vi "init queues.vi"(8 "error in (no error)":errorcluster) -> (0 "error out":errorcluster, 3 "output device queues":T1)   [LabVIEW 2016]
uses:
  data.ctl
  device/device.ctl
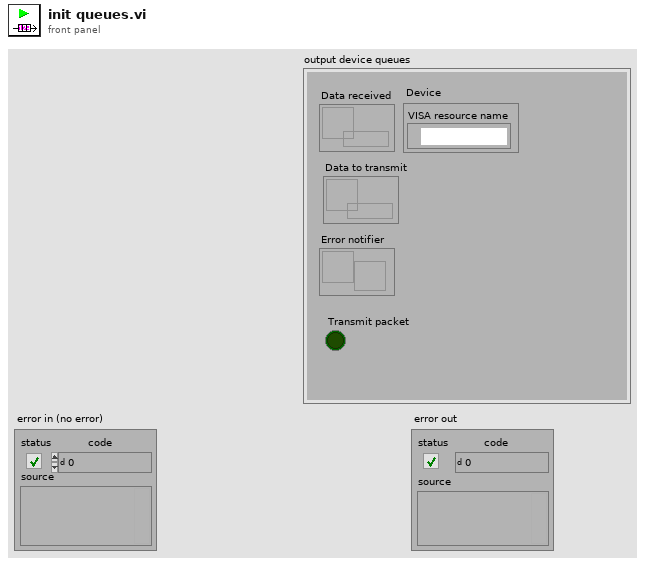
[diagram p1: front panel]
types:
  T1 = typedef "data.ctl" = cluster{"Data received":refnum<queue>, "Data to transmit":refnum<queue>, "Error notifier":refnum<notifier>, "Device":T2, "Transmit packet":bool}
  T2 = typedef "device.ctl" = cluster{"VISA resource name":refnum<visa-resource-name>}
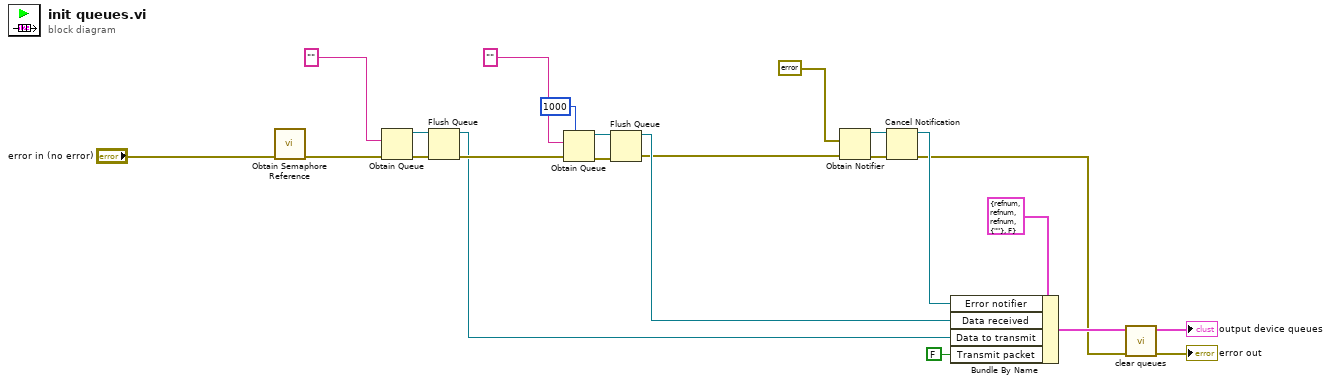
[diagram p0: block diagram]
diagram:
  n1 = call <vilib>:"Obtain Semaphore Reference.vi"("error in (no error)"="error in (no error)") -> ("error out"=w8:errorcluster)  [unwired: 4 in, 2 out]
  n2 = Obtain Queue(element data type="", error in (no error)=w8) -> (queue out=w21:refnum<queue>, error out=w20:errorcluster)  [unwired: 3 in, 1 out]
  n3 = Flush Queue(queue=w21, error in (no error)=w20) -> (queue out=w10:refnum<queue>, error out=w15:errorcluster)  [unwired: 1 out]
  n4 = Obtain Queue(max queue size (-1, unlimited)=1000, element data type="", error in (no error)=w15) -> (queue out=w16:refnum<queue>, error out=w17:errorcluster)  [unwired: 2 in, 1 out]
  n5 = Flush Queue(queue=w16, error in (no error)=w17) -> (queue out=w12:refnum<queue>, error out=w9:errorcluster)  [unwired: 1 out]
  n6 = Obtain Notifier(notification data type=errorcluster {"status"=FALSE, "code"=0, "source"=""} ("error out"), error in (no error)=w9) -> (notifier out=w19:refnum<notifier>, error out=w18:errorcluster)  [unwired: 2 in, 1 out]
  n7 = Cancel Notification(0:w19, 3:w18) -> (8:w13:refnum<notifier>, 11:w6:errorcluster)  [unwired: 1 out]
  n8 = Bundle By Name(cluster=T1 {"Data received"=refnum, "Data to transmit"=refnum, "Error notifier"=refnum, "Device"={"VISA resource name"=""}, "Transmit packet"=FALSE} ("Comm Queues"), "Error notifier"=w13, "Data received"=w12, "Data to transmit"=w10, "Transmit packet"=FALSE) -> (w7:T1)
  n9 = call "clear queues.vi"("error in (no error)"=w6, "queues"=w7) -> ("error out"=→"error out":errorcluster, "output device queues"=→"output device queues":T1)  [unwired: 8 in]
